vi "Add Thousands Separators.vi"(5 "use system decimal point (T)":bool, 7 "Thousands separator (space)":string=" ", 11 "Number as string":string) -> (3 "Number as separated string":string)   [LabVIEW 2020, in "varilib.lvlib"]
doc: "Takes number as string and separates thousands. E.g. \"1234567.1234567\" converts to \"1 234 567.123 456 7\""
uses:
  varilib.lvlib
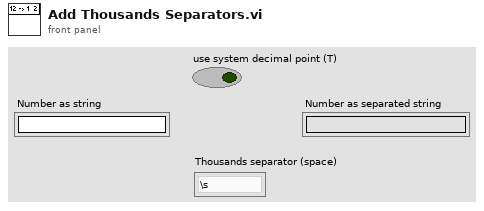
[diagram p1: front panel]
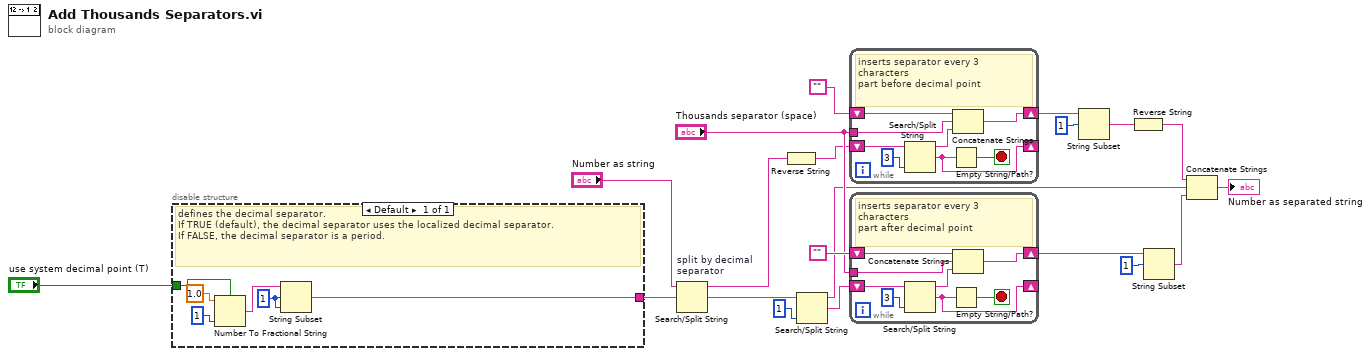
[diagram p0: block diagram]
diagram:
  n1 = disable-structure shown="Default" {
    disable-tunnel: "use system decimal point (T)" -> [w22]
    disable-tunnel: [w21] -> w7
    frame Enabled {
      w26 = 1 ("offset (0)")
      # "defines the decimal separator.\nIf TRUE (default), the decimal separator uses the localized decimal separator.\nIf FALSE, the decimal separator is a period."
      n2 = Number To Fractional String(use system decimal point (T)=w22, number=1.0, precision (6)=i16 1) -> (F-format string=w23:string)  [unwired: 1 in]
      n3 = String Subset(string=w23, offset (0)=w26, length (rest)=w26) -> (substring=w21:string)
    }
  }
  n4 = Search/Split String "split by decimal\nseparator"(string="Number as string", search string/char (-)=w7) -> (substring before match=w5:string, match + rest of string=w4:string)  [unwired: 1 in, 1 out]
  n5 = Reverse String(1:w5) -> (0:w13:string)
  n6 = Search/Split String(string=w4, offset (0)=1) -> (substring before match=w2:string, match + rest of string=w1:string)  [unwired: 1 in, 1 out]
  n7 = while {
    shift-right: [w32] -> _
    shift-left: w13 -> [w33]
    shift-right: [w28] -> w11
    shift-left: "" -> [w29]
    tunnel: "Thousands separator (space)" -> [w27]
    stop <- w31 stop-if-true
    # "inserts separator every 3 characters\npart before decimal point"
    n8 = Search/Split String(string=w33, offset (0)=3 ("length (rest)")) -> (substring before match=w30:string, match + rest of string=w32:string)  [unwired: 1 in, 1 out]
    n9 = Empty String/Path?(string/path=w32) -> (empty?=w31:bool)
    n10 = Concatenate Strings(w29, w27, w30) -> (w28:string)
  }
  n11 = while {
    shift-right: [w40] -> _
    shift-left: w1 -> [w41]
    shift-right: [w36] -> w18
    shift-left: "" -> [w37]
    tunnel: "Thousands separator (space)" -> [w35]
    stop <- w39 stop-if-true
    # "inserts separator every 3 characters\npart after decimal point"
    n12 = Search/Split String(string=w41, offset (0)=3 ("length (rest)")) -> (substring before match=w38:string, match + rest of string=w40:string)  [unwired: 1 in, 1 out]
    n13 = Empty String/Path?(string/path=w40) -> (empty?=w39:bool)
    n14 = Concatenate Strings(w37, w35, w38) -> (w36:string)
  }
  n15 = String Subset(string=w11, offset (0)=1) -> (substring=w10:string)  [unwired: 1 in]
  n16 = Reverse String(1:w10) -> (0:w9:string)
  n17 = String Subset(string=w18, offset (0)=1) -> (substring=w17:string)  [unwired: 1 in]
  n18 = Concatenate Strings(w9, w2, w17) -> (→"Number as separated string":string)
